vi "Measure_current_running_prot_loop.vi"(8 "error in (no error)":errorcluster, 11 "DAQmxTaksContainer_General in":refnum<class "DAQmxTaksContainer_General.lvclass">) -> (0 "error out":errorcluster, 1 "value":dbl, 2 "DAQmxTask en sortie":refnum<class "DAQmxTaskAICurrent_General.lvclass">, 3 "DAQmxTaksContainer_General out":refnum<class "DAQmxTaksContainer_General.lvclass">)   [LabVIEW 2020, in "DAQmxTaksContainer_General.lvclass"]
uses:
  DAQmxTaksContainer_General.lvclass
  DAQmxTaskAICurrent_General/DAQmxTaskAICurrent_General.lvclass
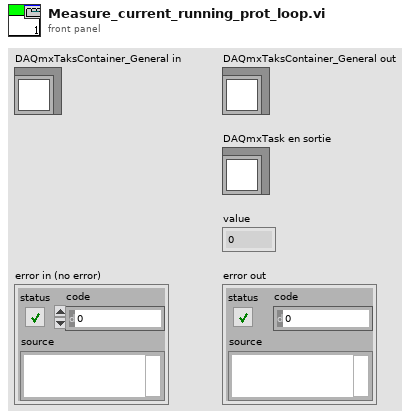
[diagram p1: front panel]
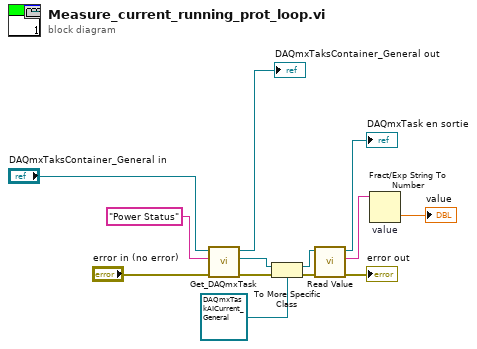
[diagram p0: block diagram]
diagram:
  n1 = call "Get_DAQmxTask.vi"("error in (no error)"="error in (no error)", "Task name"="Power Status", "DAQmxTaksContainer_General in"="DAQmxTaksContainer_General in") -> ("error out"=w8:errorcluster, "DAQmx Task"=w10:refnum<class "DAQmxTask.lvclass">, "DAQmxTaksContainer_General out"=→"DAQmxTaksContainer_General out":refnum<class "DAQmxTaksContainer_General.lvclass">)  [unwired: 6 in]
  n2 = To More Specific Class(target class=refnum<class "DAQmxTaskAICurrent_General.lvclass"> refnum ("DAQmxTaskAICurrent_General.lvclass"), reference=w10, error in=w8) -> (specific class reference=w2:refnum<class "DAQmxTaskAICurrent_General.lvclass">, error out=w3:errorcluster)
  n3 = call-dynamic "Read Value.vi"("error in (no error)"=w3, "DAQmxTask en entrée"=w2) -> ("error out"=→"error out":errorcluster, "Data string"=w1:string, "DAQmxTask en sortie"=→"DAQmxTask en sortie":refnum<class "DAQmxTaskAICurrent_General.lvclass">)  [unwired: 6 in, 1 out]
  n4 = Fract/Exp String To Number "value"(string=w1) -> (number=→"value":dbl)  [unwired: 3 in, 1 out]
